vi "Load Main.vi"(10 "Data Type DVRs":T1, 11 "Config Folder":path) -> ()   [LabVIEW 2018]
uses:
  Controls/DDS State.ctl
  <vilib>/ORNL/CSEISMIC DDS/CSEISMIC DDS Base/Data Types/SmartRelay_Measurement.ctl
  <vilib>/ORNL/CSEISMIC DDS/CSEISMIC DDS Base/Data Types/Controls/DeviceID.ctl
  Controls/Data Type DVRs.ctl
  <vilib>/ORNL/CSEISMIC DDS/CSEISMIC DDS Base/Data Types/Controls/Timestamp.ctl
  <vilib>/ORNL/CSEISMIC DDS/CSEISMIC DDS Base/Data Types/IED_Status.ctl
  da033fe5-58c0-4738-8101-30d7572e7183.vi
  e5601da1-de2b-4bec-93b1-690155eb2199.vi
  502e4aa2-f502-4312-9099-76032dc876a6.vi
  671d0d95-edd5-423e-bdac-170b3c7e1bab.vi
  94cf4db6-4932-4aea-b242-2665c68c120f.vi
  Global Variables/Stop (Global).vi
  Global Variables/DDS States (Global).vi
  Global Variables/Broadcast Topics (Global).vi
  Global Variables/Measurements (Global).vi
  Global Variables/Manual Control (Global).vi
  <vilib>/ORNL/CSEISMIC DDS/CSEISMIC DDS Base/CSEISMIC DDS.lvclass
panel:
  out "Load Data":T2
  out "DDS State":T4
  out "error out":errorcluster
  out "Error in DDS Loop":bool
  out "MicrogridID":u8
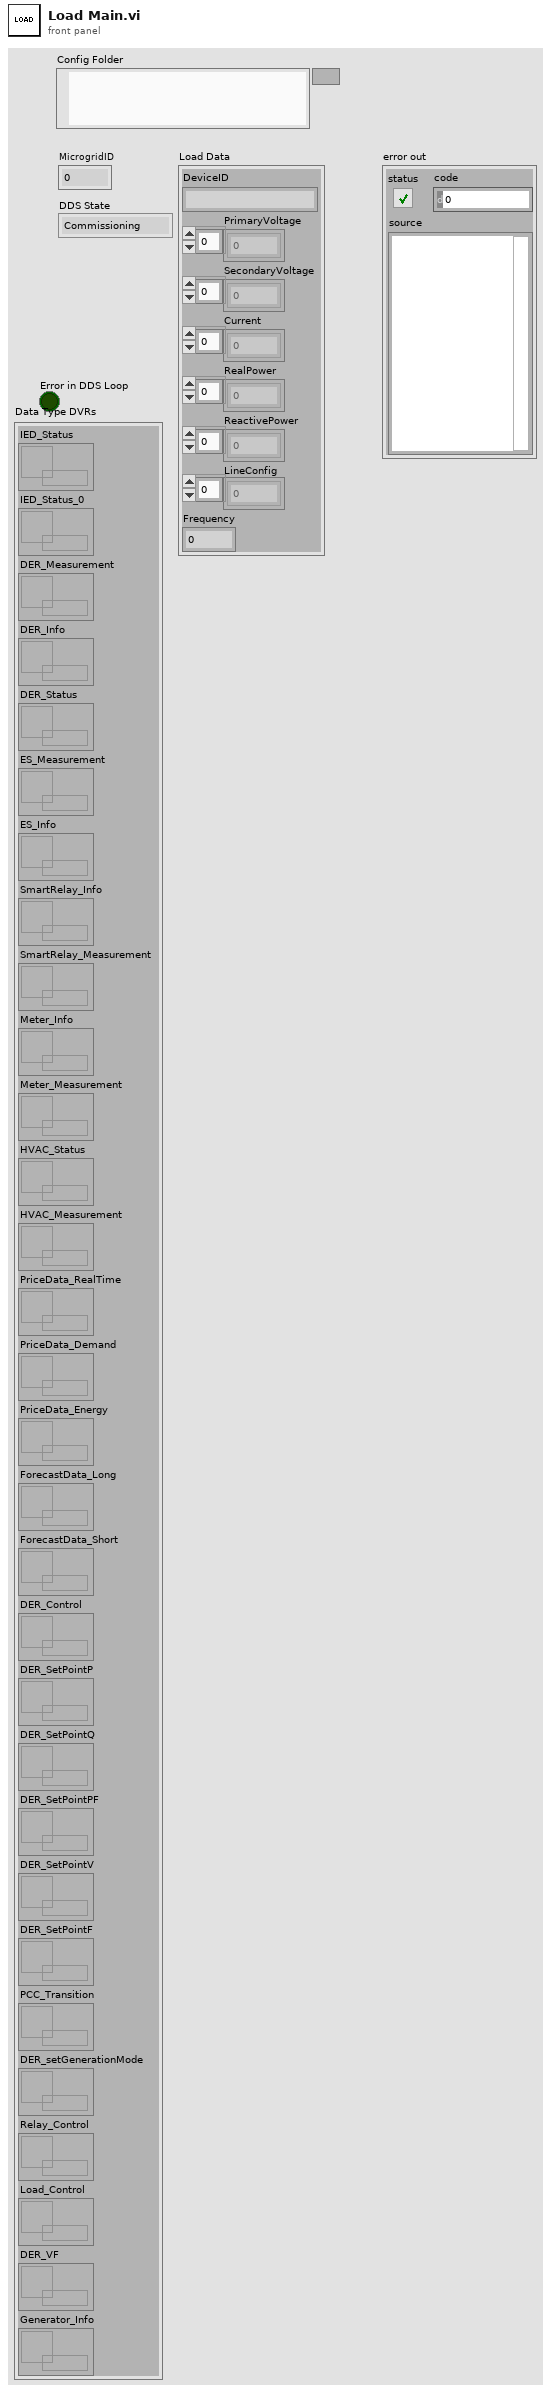
[diagram p1: front panel]
types:
  T1 = typedef "Data Type DVRs.ctl" = cluster{"IED_Status":refnum<data-value>, "IED_Status_0":refnum<data-value>, "DER_Measurement":refnum<data-value>, "DER_Info":refnum<data-value>, "DER_Status":refnum<data-value>, "ES_Measurement":refnum<data-value>, "ES_Info":refnum<data-value>, "SmartRelay_Info":refnum<data-value>, "SmartRelay_Measurement":refnum<data-value>, "Meter_Info":refnum<data-value>, "Meter_Measurement":refnum<data-value>, "HVAC_Status":refnum<data-value>, "HVAC_Measurement":refnum<data-value>, "PriceData_RealTime":refnum<data-value>, "PriceData_Demand":refnum<data-value>, "PriceData_Energy":refnum<data-value>, "ForecastData_Long":refnum<data-value>, "ForecastData_Short":refnum<data-value>, "DER_Control":refnum<data-value>, "DER_SetPointP":refnum<data-value>, "DER_SetPointQ":refnum<data-value>, "DER_SetPointPF":refnum<data-value>, "DER_SetPointV":refnum<data-value>, "DER_SetPointF":refnum<data-value>, "PCC_Transition":refnum<data-value>, "DER_setGenerationMode":refnum<data-value>, "Relay_Control":refnum<data-value>, "Load_Control":refnum<data-value>, "DER_VF":refnum<data-value>, "Generator_Info":refnum<data-value>}
  T2 = typedef "CSEISMIC DDS.lvlib/CSEISMIC DDS.lvclass/SmartRelay_Measurement.ctl" = cluster{"DeviceID":T3, "PrimaryVoltage":dbl[], "SecondaryVoltage":dbl[], "Current":dbl[], "RealPower":dbl[], "ReactivePower":dbl[], "LineConfig":u8[], "Frequency":dbl}
  T3 = typedef "CSEISMIC DDS.lvlib/CSEISMIC DDS.lvclass/DeviceID.ctl" = string
  T4 = typedef "DDS State.ctl" = enum16{"Commissioning", "CheckID", "InitDDS", "ReadDDS", "WriteDDS", "CheckClose", "Close", "Shutdown"}
  T5 = typedef "CSEISMIC DDS.lvlib/CSEISMIC DDS.lvclass/SmartRelay_Info.ctl" = cluster{"DeviceID":T3, "LineConfig":u8[], "NominalVoltage(V)":dbl}
  T6 = typedef "CSEISMIC DDS.lvlib/CSEISMIC DDS.lvclass/IED_Status.ctl" = cluster{"DeviceID":T3, "Timestamp":T7, "MicrogridID":u8, "Active":bool, "Inactive":bool, "Error":i32, "Fault":bool, "ErrorString":string}
  T7 = typedef "CSEISMIC DDS.lvlib/CSEISMIC DDS.lvclass/Timestamp.ctl" = cluster{"Seconds":u64, "Remainder":u64}
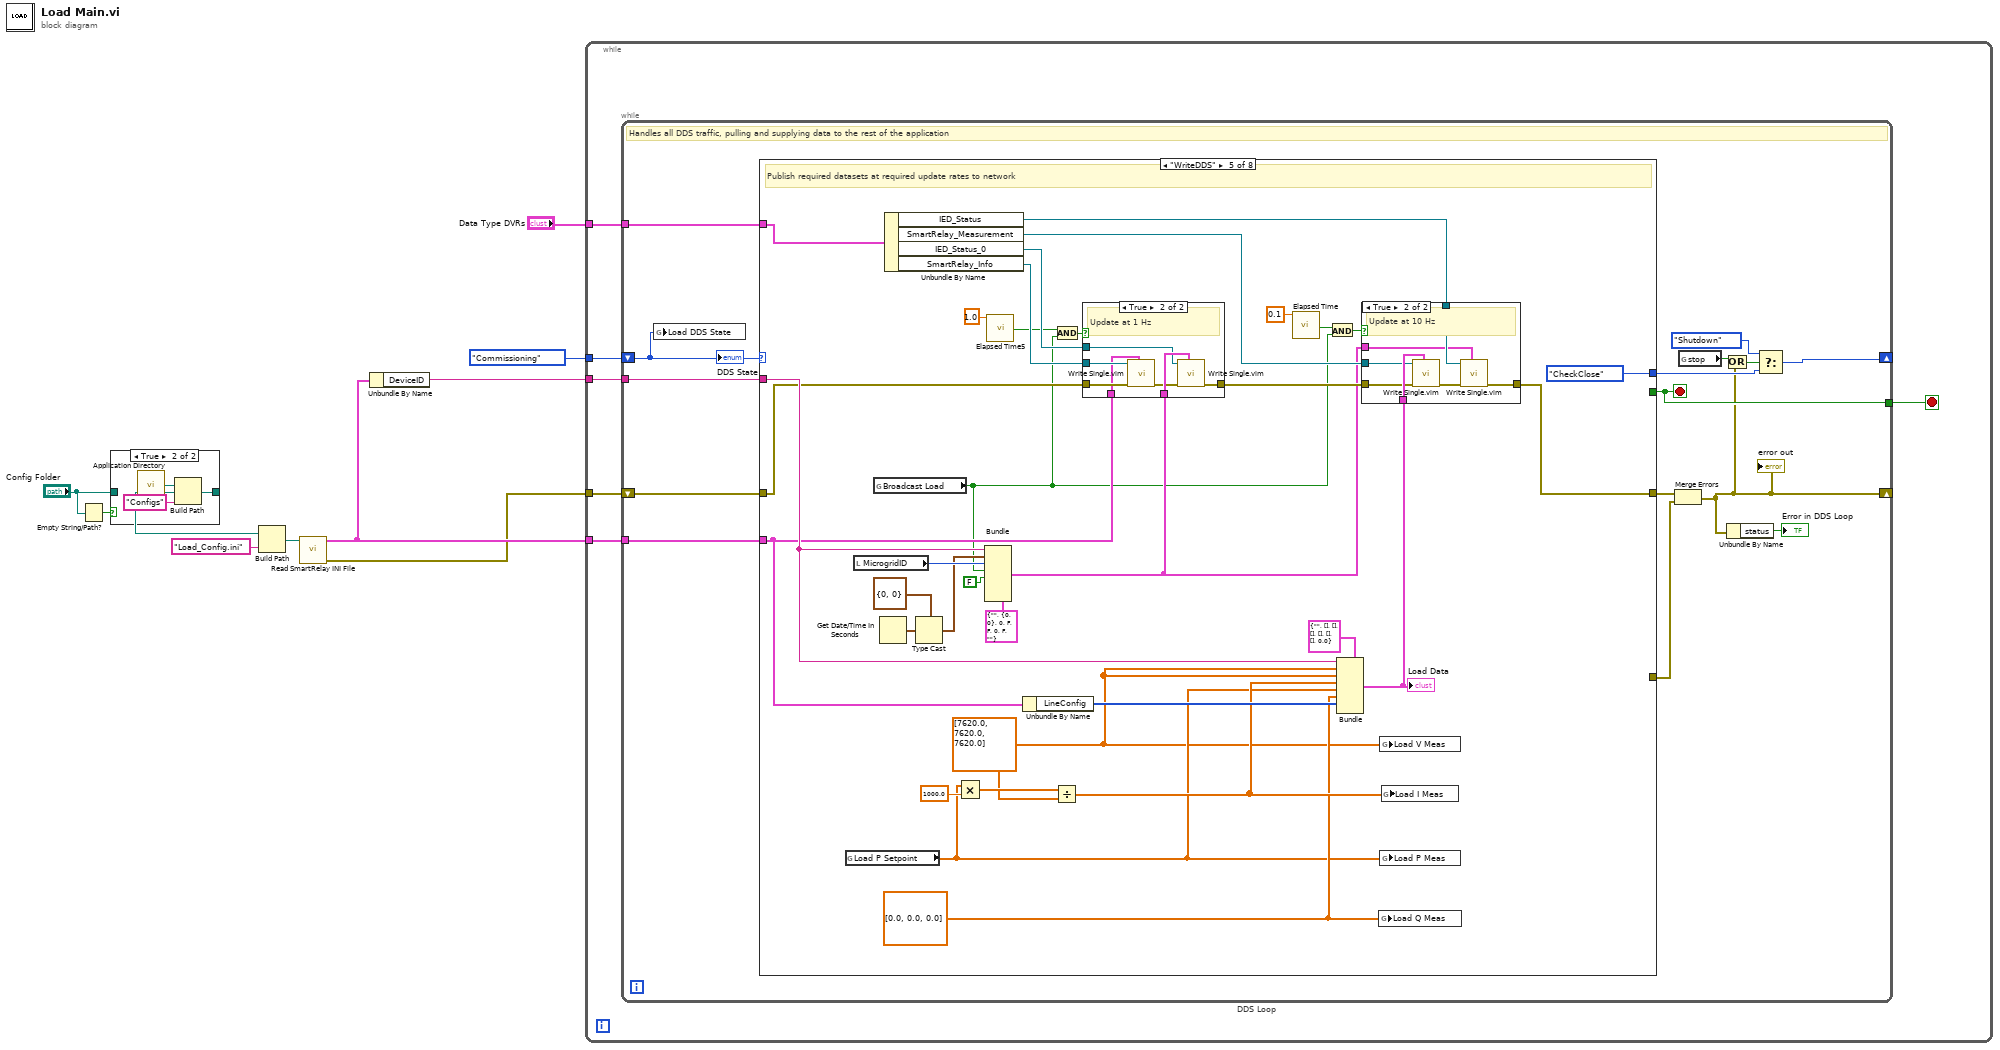
[diagram p0: block diagram]
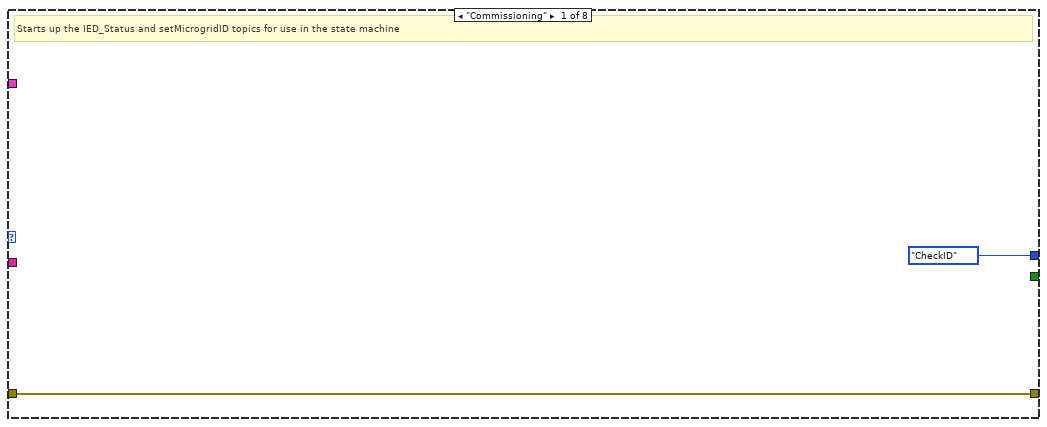
[diagram p2: hidden frame]
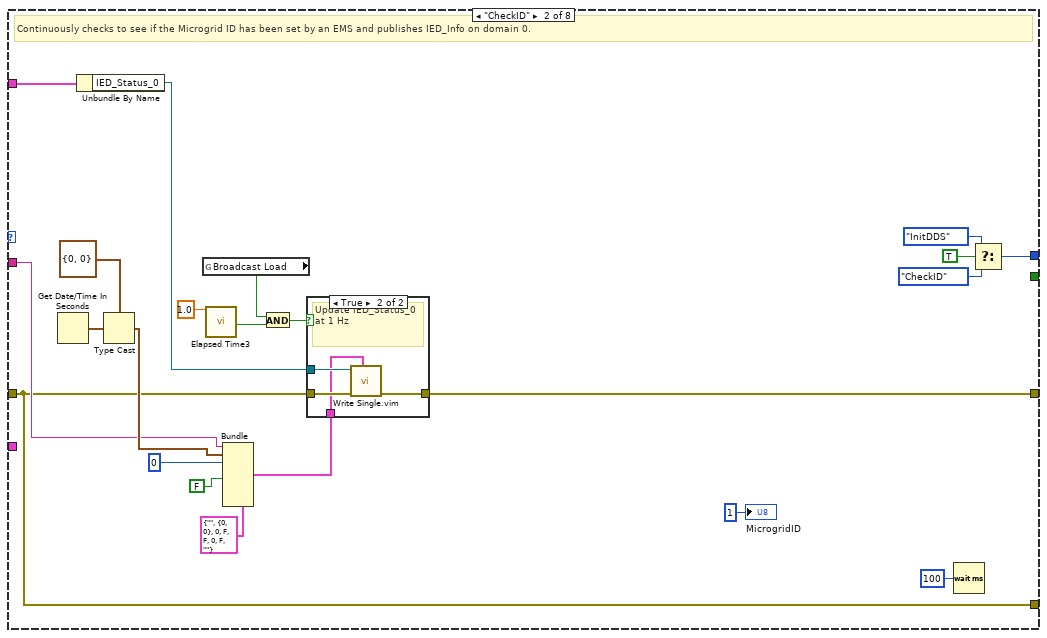
[diagram p3: hidden frame]
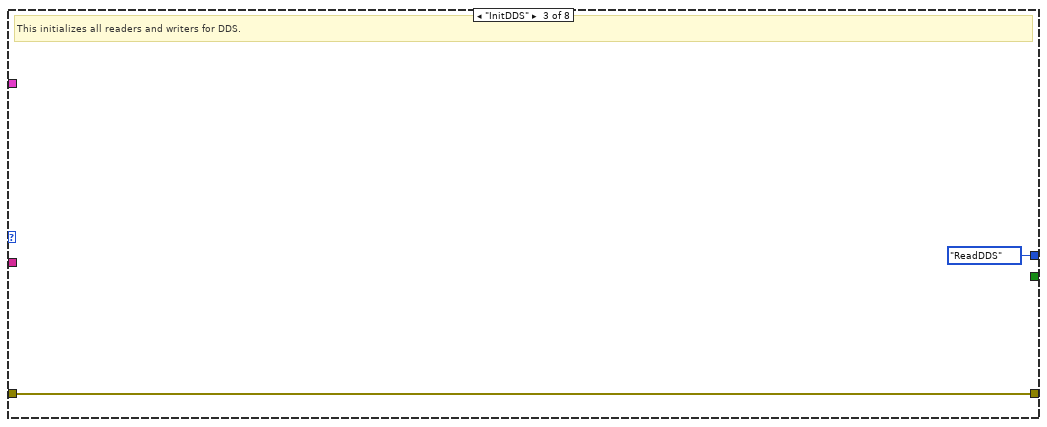
[diagram p5: hidden frame]
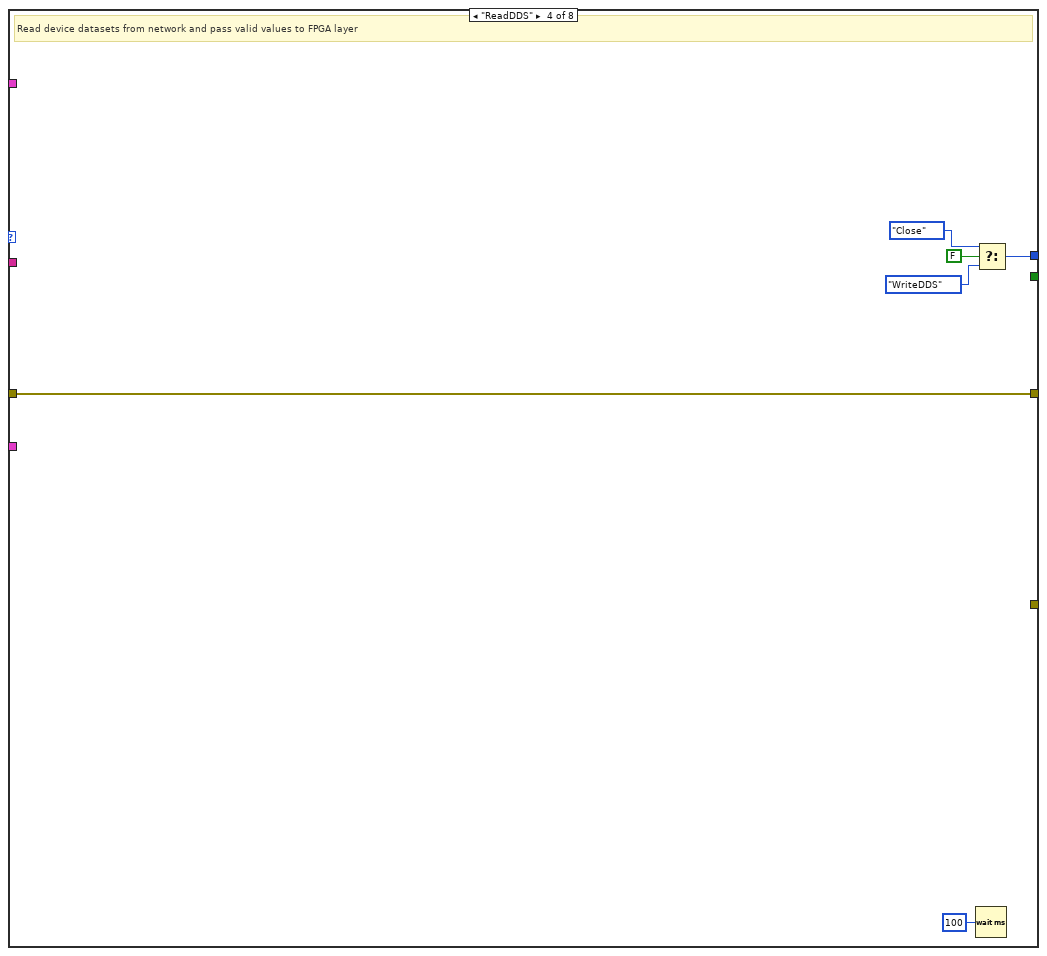
[diagram p6: hidden frame]
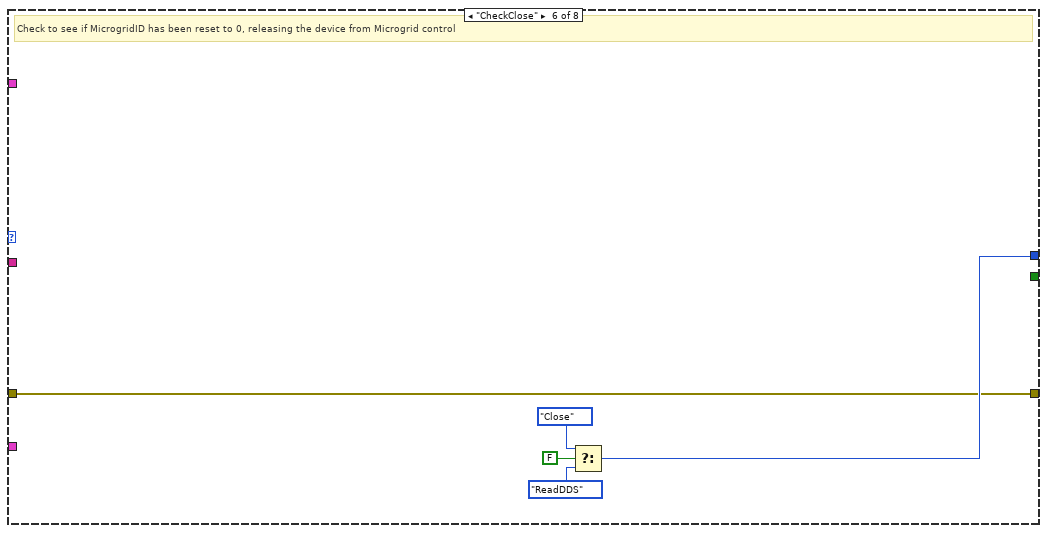
[diagram p9: hidden frame]
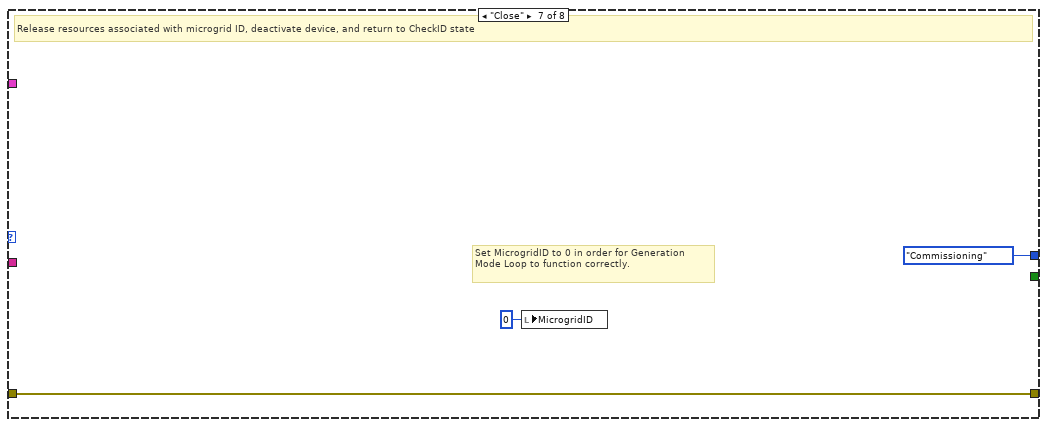
[diagram p10: hidden frame]
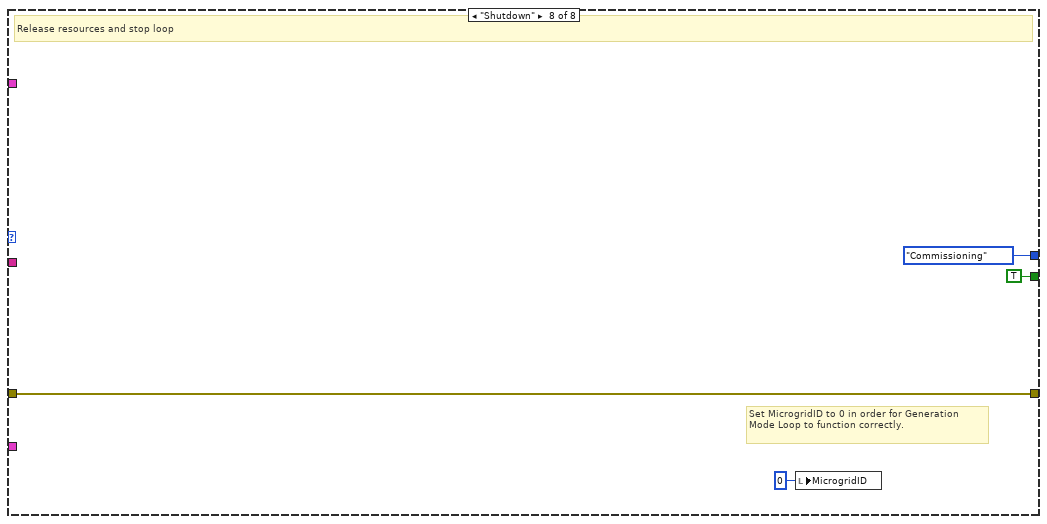
[diagram p11: hidden frame]
diagram:
  n1 = Empty String/Path?(string/path="Config Folder") -> (empty?=w4:bool)
  n2 = case shown="True" w4 {
    tunnel: [w11 w12] -> w2
    tunnel: "Config Folder" -> [w11 _]
    frame False {
    }
    frame True {
      n3 = call <vilib>:"Application Directory.vi"() -> ("Application Directory"=w14:path)
      n4 = Build Path(base path=w14, name or relative path="Configs") -> (appended path=w12:path)
    }
  }
  n5 = Build Path(base path=w2, name or relative path="Load_Config.ini") -> (appended path=w5:path)
  n6 = call "Read SmartRelay INI File.vi"("Path"=w5) -> ("error out"=w7:errorcluster, "SmartRelay_Info"=w9:T5)  [unwired: 8 in, 1 out]
  n7 = Unbundle By Name(w9) -> ("DeviceID"=w8:T3)
  n8 = while {
    tunnel: DDS_State."Commissioning" -> [w20]
    tunnel: w7 -> [w19]
    tunnel: w8 -> [w18]
    tunnel: w9 -> [w17]
    tunnel: "Data Type DVRs" -> [w15]
    stop <- w16 stop-if-true
    n9 = while "DDS Loop" {
      shift-right: [w32] -> _
      shift-left: w20 -> [w21]
      tunnel: w18 -> [w35]
      shift-right: [w24] -> _
      shift-left: w19 -> [w34]
      tunnel: w17 -> [w33]
      tunnel: [w27] -> w16
      tunnel: w15 -> [w26]
      stop <- w27 stop-if-true
      # "Handles all DDS traffic, pulling and supplying data to the rest of the application"
      n10 = global write "DDS States (Global).vi" "Load DDS State"(w21) -> ()
      n11 = case shown="\"WriteDDS\"" w21 {
        tunnel: [DDS_State."CheckID" w56 DDS_State."ReadDDS" w70 DDS_State."CheckClose" w125 DDS_State."Commissioning" ("f") DDS_State."Commissioning" ("f")] -> w31
        tunnel: [w36 w43 w65 w68 w86 w124 w129 w131] -> w25
        tunnel: w35 -> [_ w48 _ _ w105 _ _ _]
        tunnel: w34 -> [w36 w44 w65 w68 w87 w124 w129 w131]
        tunnel: w33 -> [_ _ _ _ w83 _ _ _]
        tunnel: [_ _ _ _ _ _ _ TRUE] -> w27
        tunnel: w26 -> [_ w47 _ _ w85 _ _ _]
        tunnel: [_ w44 _ _ _ _ _ _] -> w23
        frame "Commissioning" {
          # "Starts up the IED_Status and setMicrogridID topics for use in the state machine"
        }
        frame "CheckID" {
          # "Continuously checks to see if the Microgrid ID has been set by an EMS and publishes IED_Info on domain 0."
          n12 = Get Date/Time In Seconds() -> (seconds since 1Jan1904=w52:timestamp)
          n13 = Unbundle By Name(w47) -> ("IED_Status_0"=w46:refnum<data-value>)
          n14 = Type Cast(type=T7 {"Seconds"=0, "Remainder"=0} ("Timestamp"), x=w52) -> (*(type *) &x=w51:T7)
          n15 = global read "Broadcast Topics (Global).vi" "Broadcast Load"() -> (w38:bool)
          n16 = call "Elapsed Time3"("Time Target (s)"=1.0) -> ("Time has Elapsed"=w39:bool)  [unwired: 11 in, 7 out]
          n17 = Bundle(cluster=T6 {"DeviceID"="", "Timestamp"={"Seconds"=0, "Remainder"=0}, "MicrogridID"=0, "Active"=FALSE, "Inactive"=FALSE, "Error"=0, "Fault"=FALSE, "ErrorString"=""} ("output cluster"), "DeviceID"=w48, "Timestamp"=w51, "MicrogridID"=u8 0, "Inactive"=FALSE ("Active")) -> (w45:T6)  [unwired: 4 in]
          n18 = And(x=w38, y=w39) -> (x .and. y?=w40:bool)
          n19 = case shown="True" w40 {
            tunnel: w45 -> [_ w61]
            tunnel: [w60 w62] -> w43
            tunnel: w44 -> [w60 w63]
            tunnel: w46 -> [_ w64]
            frame False {
            }
            frame True {
              # "Update IED_Status_0 at 1 Hz"
              n20 = call "Write Single.vim"("Data Element"=w61, "error in"=w63, "Data DVR"=w64) -> ("dup error out"=w62:errorcluster)  [unwired: 8 in]
            }
          }
          n21 = Wait (ms)(milliseconds to wait=u32 100) -> ()  [unwired: 1 out]
          n22 = Select(t=DDS_State."InitDDS", s=TRUE, f=DDS_State."CheckID") -> (s? t:f=w56:T4)
          "MicrogridID" <- u8 1 ("MicrogridID")
        }
        frame "InitDDS" {
          # "This initializes all readers and writers for DDS."
        }
        frame "ReadDDS" {
          # "Read device datasets from network and pass valid values to FPGA layer"
          n23 = Wait (ms)(milliseconds to wait=u32 100) -> ()  [unwired: 1 out]
          n24 = Select(t=DDS_State."Close", s=FALSE, f=DDS_State."WriteDDS") -> (s? t:f=w70:T4)
        }
        frame "WriteDDS" {
          w79 = dbl[] [0.0, 0.0, 0.0]
          w73 = dbl[] [7620.0, 7620.0, 7620.0]
          # "Publish required datasets at required update rates to network"
          n25 = global read "Manual Control (Global).vi" "Load P Setpoint"() -> (w74:dbl[])
          n26 = local read "MicrogridID"() -> (w104:u8)
          n27 = global read "Broadcast Topics (Global).vi" "Broadcast Load"() -> (w75:bool)
          n28 = Get Date/Time In Seconds() -> (seconds since 1Jan1904=w102:timestamp)
          n29 = Unbundle By Name(w85) -> ("IED_Status"=w84:refnum<data-value>, "SmartRelay_Measurement"=w94:refnum<data-value>, "IED_Status_0"=w93:refnum<data-value>, "SmartRelay_Info"=w92:refnum<data-value>)
          n30 = Type Cast(type=T7 {"Seconds"=0, "Remainder"=0} ("Timestamp"), x=w102) -> (*(type *) &x=w101:T7)
          n31 = Multiply(x=w74, y=1000.0) -> (x*y=w95:dbl[])
          n32 = Bundle(cluster=T6 {"DeviceID"="", "Timestamp"={"Seconds"=0, "Remainder"=0}, "MicrogridID"=0, "Active"=FALSE, "Inactive"=FALSE, "Error"=0, "Fault"=FALSE, "ErrorString"=""} ("IED_Status"), "DeviceID"=w105, "Timestamp"=w101, "MicrogridID"=w104, "Active"=w75, "Inactive"=FALSE ("Active")) -> (w82:T6)  [unwired: 3 in]
          n33 = call "Elapsed Time5"("Time Target (s)"=1.0) -> ("Time has Elapsed"=w77:bool)  [unwired: 11 in, 7 out]
          n34 = Unbundle By Name(w83) -> ("LineConfig"=w98:u8[])
          n35 = Divide(x=w95, y=w73) -> (x/y=w80:dbl[])
          n36 = And(x=w77, y=w75) -> (x .and. y?=w78:bool)
          n37 = case shown="True" w78 {
            tunnel: w87 -> [w115 w122]
            tunnel: [w115 w118] -> w88
            tunnel: w82 -> [_ w120]
            tunnel: w83 -> [_ w116]
            tunnel: w92 -> [_ w121]
            tunnel: w93 -> [_ w119]
            frame False {
            }
            frame True {
              # "Update at 1 Hz"
              n38 = call "Write Single.vim"("Data Element"=w116, "error in"=w122, "Data DVR"=w121) -> ("dup error out"=w117:errorcluster)  [unwired: 8 in]
              n39 = call "Write Single.vim"("Data Element"=w120, "error in"=w117, "Data DVR"=w119) -> ("dup error out"=w118:errorcluster)  [unwired: 8 in]
            }
          }
          n40 = call "Elapsed Time"("Time Target (s)"=0.1) -> ("Time has Elapsed"=w90:bool)  [unwired: 11 in, 7 out]
          n41 = And(x=w90, y=w75) -> (x .and. y?=w76:bool)
          n42 = Bundle(cluster=T2 {"DeviceID"="", "PrimaryVoltage"=[], "SecondaryVoltage"=[], "Current"=[], "RealPower"=[], "ReactivePower"=[], "LineConfig"=[], "Frequency"=0.0} ("SmartRelay_Measurement"), "DeviceID"=w105, "PrimaryVoltage"=w73, "SecondaryVoltage"=w73, "Current"=w80, "RealPower"=w74, "ReactivePower"=w79, "LineConfig"=w98) -> (w81:T2)  [unwired: 1 in]
          "Load Data" <- w81
          n43 = case shown="True" w76 {
            tunnel: w88 -> [w107 w113]
            tunnel: w81 -> [_ w114]
            tunnel: [w107 w110] -> w86
            tunnel: w94 -> [_ w112]
            tunnel: w84 -> [_ w109]
            tunnel: w82 -> [_ w108]
            frame False {
            }
            frame True {
              # "Update at 10 Hz"
              n44 = call "Write Single.vim"("Data Element"=w114, "error in"=w113, "Data DVR"=w112) -> ("dup error out"=w111:errorcluster)  [unwired: 8 in]
              n45 = call "Write Single.vim"("Data Element"=w108, "error in"=w111, "Data DVR"=w109) -> ("dup error out"=w110:errorcluster)  [unwired: 8 in]
            }
          }
          n46 = global write "Measurements (Global).vi" "Load Q Meas"(w79) -> ()
          n47 = global write "Measurements (Global).vi" "Load V Meas"(w73) -> ()
          n48 = global write "Measurements (Global).vi" "Load P Meas"(w74) -> ()
          n49 = global write "Measurements (Global).vi" "Load I Meas"(w80) -> ()
        }
        frame "CheckClose" {
          # "Check to see if MicrogridID has been reset to 0, releasing the device from Microgrid control"
          n50 = Select(t=DDS_State."Close", s=FALSE, f=DDS_State."ReadDDS") -> (s? t:f=w125:T4)
        }
        frame "Close" {
          # "Set MicrogridID to 0 in order for Generation Mode Loop to function correctly."
          # "Release resources associated with microgrid ID, deactivate device, and return to CheckID state"
          n51 = local write "MicrogridID"(u8 0 ("MicrogridID")) -> ()
        }
        frame "Shutdown" {
          # "Set MicrogridID to 0 in order for Generation Mode Loop to function correctly."
          # "Release resources and stop loop"
          n52 = local write "MicrogridID"(u8 0 ("MicrogridID")) -> ()
        }
      }
      n53 = Merge Errors(w25, w23) -> (w24:errorcluster)
      "error out" <- w24
      n54 = global read "Stop (Global).vi" "stop"() -> (w22:bool)
      n55 = Or(x=w22, y=w24) -> (x .or. y?=w29:bool)
      n56 = Unbundle By Name(w24) -> ("status"=→"Error in DDS Loop":bool)
      n57 = Select(t=DDS_State."Shutdown", s=w29, f=w31) -> (s? t:f=w32:T4)
      "DDS State" <- w21
    }
  }
